vi "add_analysis_data.vi"(8 "error in (no error)":errorcluster, 10 "single analysis data":string[](array[string]), 11 "Analysis in":refnum<class "Analysis.lvclass">) -> (0 "error out":errorcluster, 3 "Analysis out":refnum<class "Analysis.lvclass">)   [LabVIEW 2018, in "Analysis.lvclass"]
doc: "adds data to the analysis data arrray (isotope_name,time, signal).\nThe full array is 3-dim array in order to store multiple sets of data (e.g. analysis results for each isotope).\n\nInput is a 1-dim array that holds one single point of a scan (isotope_name, time, signal)"
uses:
  Analysis.lvclass
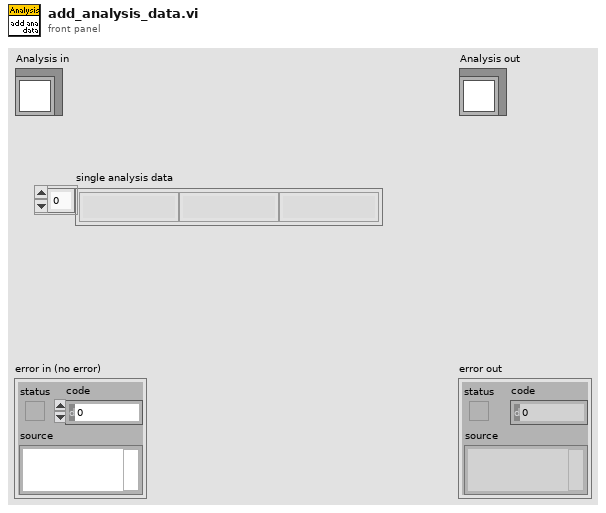
[diagram p1: front panel]
types:
  T1 = typedef "AnalysisDataArray.ctl" = cluster{"analysis data":string[][]}[]
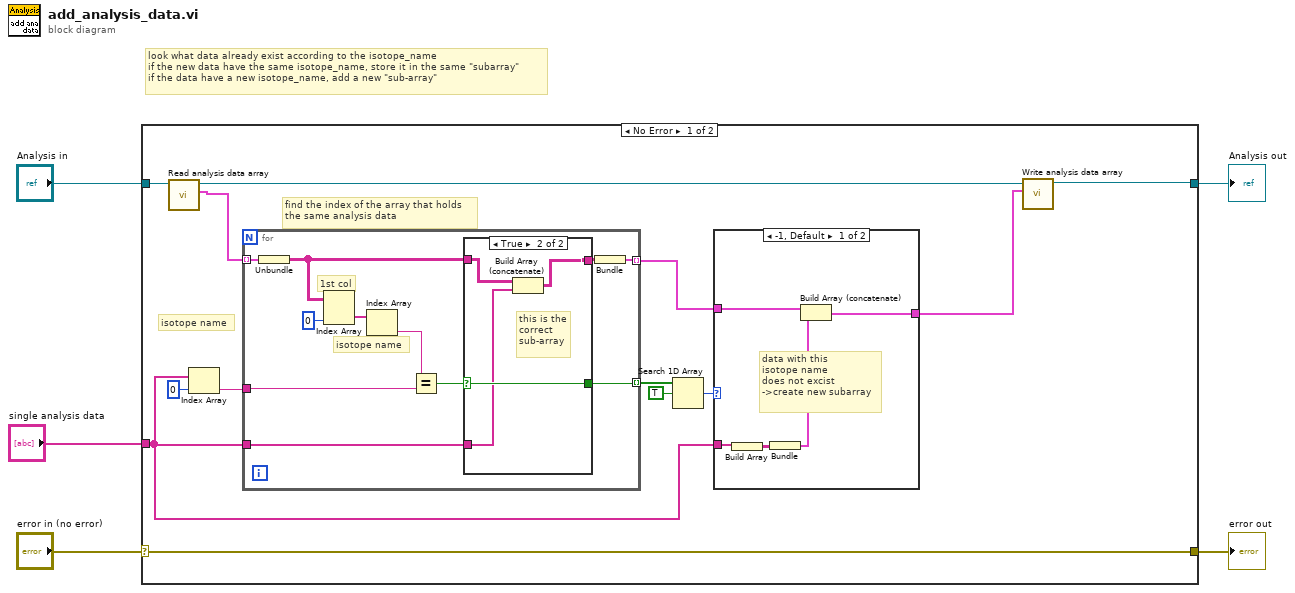
[diagram p0: block diagram]
diagram:
  # "look what data already exist according to the isotope_name\nif the new data have the same isotope_name, store it in the same \"subarray\"\nif the data have a new isotope_name, add a new \"sub-array\""
  n1 = case shown="No Error" "error in (no error)" {
    selector: "error in (no error)" -> [w18 w43]
    tunnel: [w18 w43] -> w4
    tunnel: [w15 w42] -> w2
    tunnel: "Analysis in" -> [w17 w42]
    tunnel: "single analysis data" -> [w7 _]
    frame No Error {
      # "find the index of the array that holds\nthe same analysis data"
      # "isotope name"
      n2 = call-dynamic "Read analysis data array.vi"("Analysis in"=w17) -> ("analysis data array"=w8:T1, "Analysis out"=w16:refnum<class "Analysis.lvclass">)  [unwired: 8 in, 1 out]
      n3 = Index Array(array=w7, index=0) -> (element=w12:string)
      n4 = for {
        tunnel: w8 -> [w28] mode=indexing
        tunnel: w12 -> [w32]
        tunnel: [w29] -> w13 mode=indexing
        tunnel: [w26] -> w9 mode=indexing
        tunnel: w7 -> [w31]
        # "isotope name"
        # "1st col"
        n5 = Unbundle(w28) -> ("analysis data"=w27:string[][])
        n6 = Index Array(array=w27, index (col)=0 ("disabled index (col)")) -> (element=w34:string[])  [unwired: 1 in]
        n7 = Index Array(array=w34) -> (element=w33:string)  [unwired: 1 in]
        n8 = Equal?(x=w33, y=w32) -> (x = y?=w30:bool)
        n9 = case shown="True" w30 {
          selector: w30 -> [w37 w41]
          tunnel: w31 -> [_ w38]
          tunnel: [w37 w41] -> w29
          tunnel: w27 -> [w36 w40]
          tunnel: [w36 w39] -> w25
          frame False {
            # "not the right\nsub-array"
          }
          frame True {
            # "this is the\ncorrect\nsub-array"
            n10 = Build Array (concatenate)(w40, w38) -> (w39:string[][])
          }
        }
        n11 = Bundle("analysis data"=w25) -> (w26:cluster{"analysis data":string[][]})  [unwired: 1 in]
      }
      n12 = Search 1D Array(1D array=w13, element=TRUE) -> (index of element=w10:i32)  [unwired: 1 in]
      n13 = case shown="-1, Default" w10 {
        tunnel: w9 -> [w21 w24]
        tunnel: w7 -> [w23 _]
        tunnel: [w22 w24] -> w6
        frame -1, Default {
          # "data with this\nisotope name\ndoes not excist\n->create new subarray"
          n14 = Build Array(w23) -> (w20:string[][])
          n15 = Bundle(w20) -> (w19:cluster{string[][]})  [unwired: 1 in]
          n16 = Build Array (concatenate)(w21, w19) -> (w22:cluster{"analysis data":string[][]}[])
        }
        frame 0.. {
          # "all fine, data have been\ninserted already"
        }
      }
      n17 = call-dynamic "Write analysis data array.vi"("analysis data array"=w6, "Analysis in"=w16) -> ("Analysis out"=w15:refnum<class "Analysis.lvclass">)  [unwired: 8 in, 1 out]
    }
    frame Error {
    }
  }
  "error out" <- w4
  "Analysis out" <- w2
